vi "Get Displacement.vi"(8 "error in (no error)":errorcluster, 11 "Displacement Sensor in":refnum<class "DispSnsr.lvclass">) -> (0 "error out":errorcluster, 2 "Displacement":dbl, 3 "Displacement Sensor out":refnum<class "DispSnsr.lvclass">)   [LabVIEW 2016, in "Hardware.lvlib" / "Displacement Sensor.lvlib" / "DispSnsr.lvclass"]
uses:
  <userlib>/Common Components/Hardware/Displacement Sensor/DispSnsr/DispSnsr.lvclass
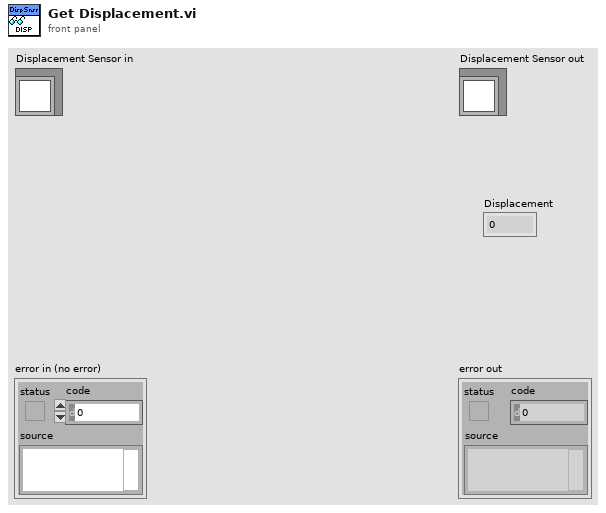
[diagram p1: front panel]
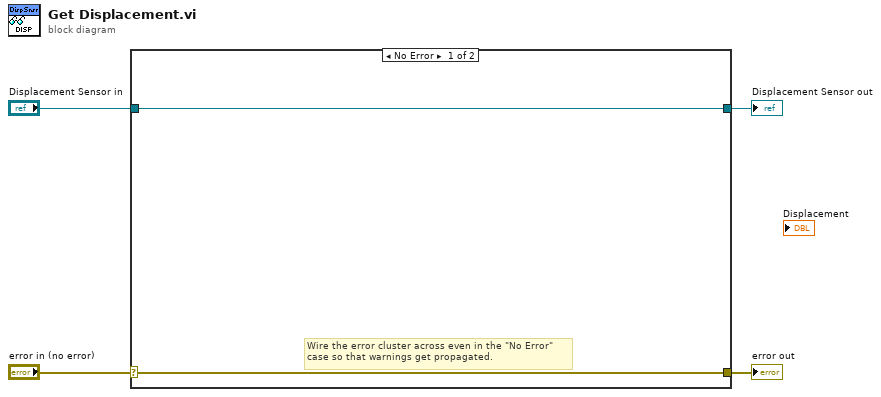
[diagram p0: block diagram]
diagram:
  n1 = case shown="No Error" "error in (no error)" {
    selector: "error in (no error)" -> [w5 w8]
    tunnel: [w5 w8] -> w3
    tunnel: [w6 w7] -> w1
    tunnel: "Displacement Sensor in" -> [w6 w7]
    frame No Error {
      # "Wire the error cluster across even in the \"No Error\"\ncase so that warnings get propagated."
    }
    frame Error {
    }
  }
  "error out" <- w3
  "Displacement Sensor out" <- w1
